vi "4 probe data v1.1.vi"() -> ()   [LabVIEW 2014]
uses:
  <vilib>/Analysis/baseanly.llb/Mean (DBL).vi
  <vilib>/MakerHub/LINX/Public/Peripherals/Analog/Analog Read 1 Chan.vi
  <instrlib>/Tektronix TDS 200 1000 2000 Series/Tektronix TDS 200 1000 2000 Series.lvlib
  <vilib>/MakerHub/LINX/LMH-LINX.lvlib
  <vilib>/Analysis/NI_AALBase.lvlib
panel:
  out "Data":string
  in  "Save File":path=path "c:/myfile.txt"
  out "Wavelength-Intensity Graph":cluster{"Y":dbl[], "Y":dbl[]}[](graph)
  out "Ch1 2":waveform(dbl)[](graph)
  out "Ch2 2":waveform(dbl)[](graph)
  out "Ch3 2":waveform(dbl)[](graph)
  out "Ch4 2":waveform(dbl)[](graph)
  out "Ch1":dbl
  out "Ch2":dbl
  out "Ch3":dbl
  out "Ch4":dbl
  out "Analog Data 0":dbl(graph)
  out "Loop Rate (Hz)":u32
  out "Analog Data 1":dbl(graph)
  out "Analog Data 2":dbl(graph)
  out "Analog Data 3":dbl(graph)
  out "Analog Data 4":dbl(graph)
  out "Numeric":dbl
  in  "AI Channel 4":u8
  in  "AI Channel 3":u8
  in  "AI Channel 2":u8
  in  "AI Channel 1":u8
  in  "AI Channel 0":u8
  in  "Serial Port":refnum<visa-resource-name>
  in  "Channel 4 (3: Channel 4)":u16(ring) items=["Channel 1", "Channel 2", "Channel 3", "Channel 4", "Math", "Reference A", "Reference B", "Reference C", "Reference D"]
  in  "Probe Attenuation 4 (0.1)":dbl=10.0
  in  "Vertical Coupling 4 (1: DC)":u16(ring)=1 items=["AC", "DC", "Ground"]
  in  "Channel 3 (2: Channel 3)":u16(ring) items=["Channel 1", "Channel 2", "Channel 3", "Channel 4", "Math", "Reference A", "Reference B", "Reference C", "Reference D"]
  in  "Probe Attenuation 3 (0.1)":dbl=10.0
  in  "Vertical Coupling 3 (1: DC)":u16(ring)=1 items=["AC", "DC", "Ground"]
  in  "Channel 2 (1: Channel 2)":u16(ring)=1 items=["Channel 1", "Channel 2", "Channel 3", "Channel 4", "Math", "Reference A", "Reference B", "Reference C", "Reference D"]
  in  "Channel 1 (0: Channel 1)":u16(ring) items=["Channel 1", "Channel 2", "Channel 3", "Channel 4", "Math", "Reference A", "Reference B", "Reference C", "Reference D"]
  in  "Serial Configuration":T1={"Baud Rate"=9600, "Parity"=0, "Stop Bits"=10, "Flow Control"=2} {"Flow Control" items=["None", "XON/XOFF", "RTS/CTS", "XON/XOFF & RTS/CTS", "DTR/DSR", "XON/XOFF & DTR/DSR"]; "Stop Bits" items=["1.0"=10, "1.5"=15, "2.0"=20]; "Parity" items=["None", "Odd", "Even", "Mark", "Space"]; "Baud Rate" items=["300"=300, "600"=600, "1200"=1200, "2400"=2400, "4800"=4800, "9600"=9600, "19200"=19200]}
  in  "Probe Attenuation 2 (0.1)":dbl=1.0
  in  "Vertical Coupling 2 (1: DC)":u16(ring)=1 items=["AC", "DC", "Ground"]
  in  "Probe Attenuation 1 (0.1)":dbl=10.0
  in  "Vertical Coupling 1 (1: DC)":u16(ring)=1 items=["AC", "DC", "Ground"]
  in  "Timeout (10000 ms)":u32=10000
  in  "VISA resource name":refnum<visa-resource-name>
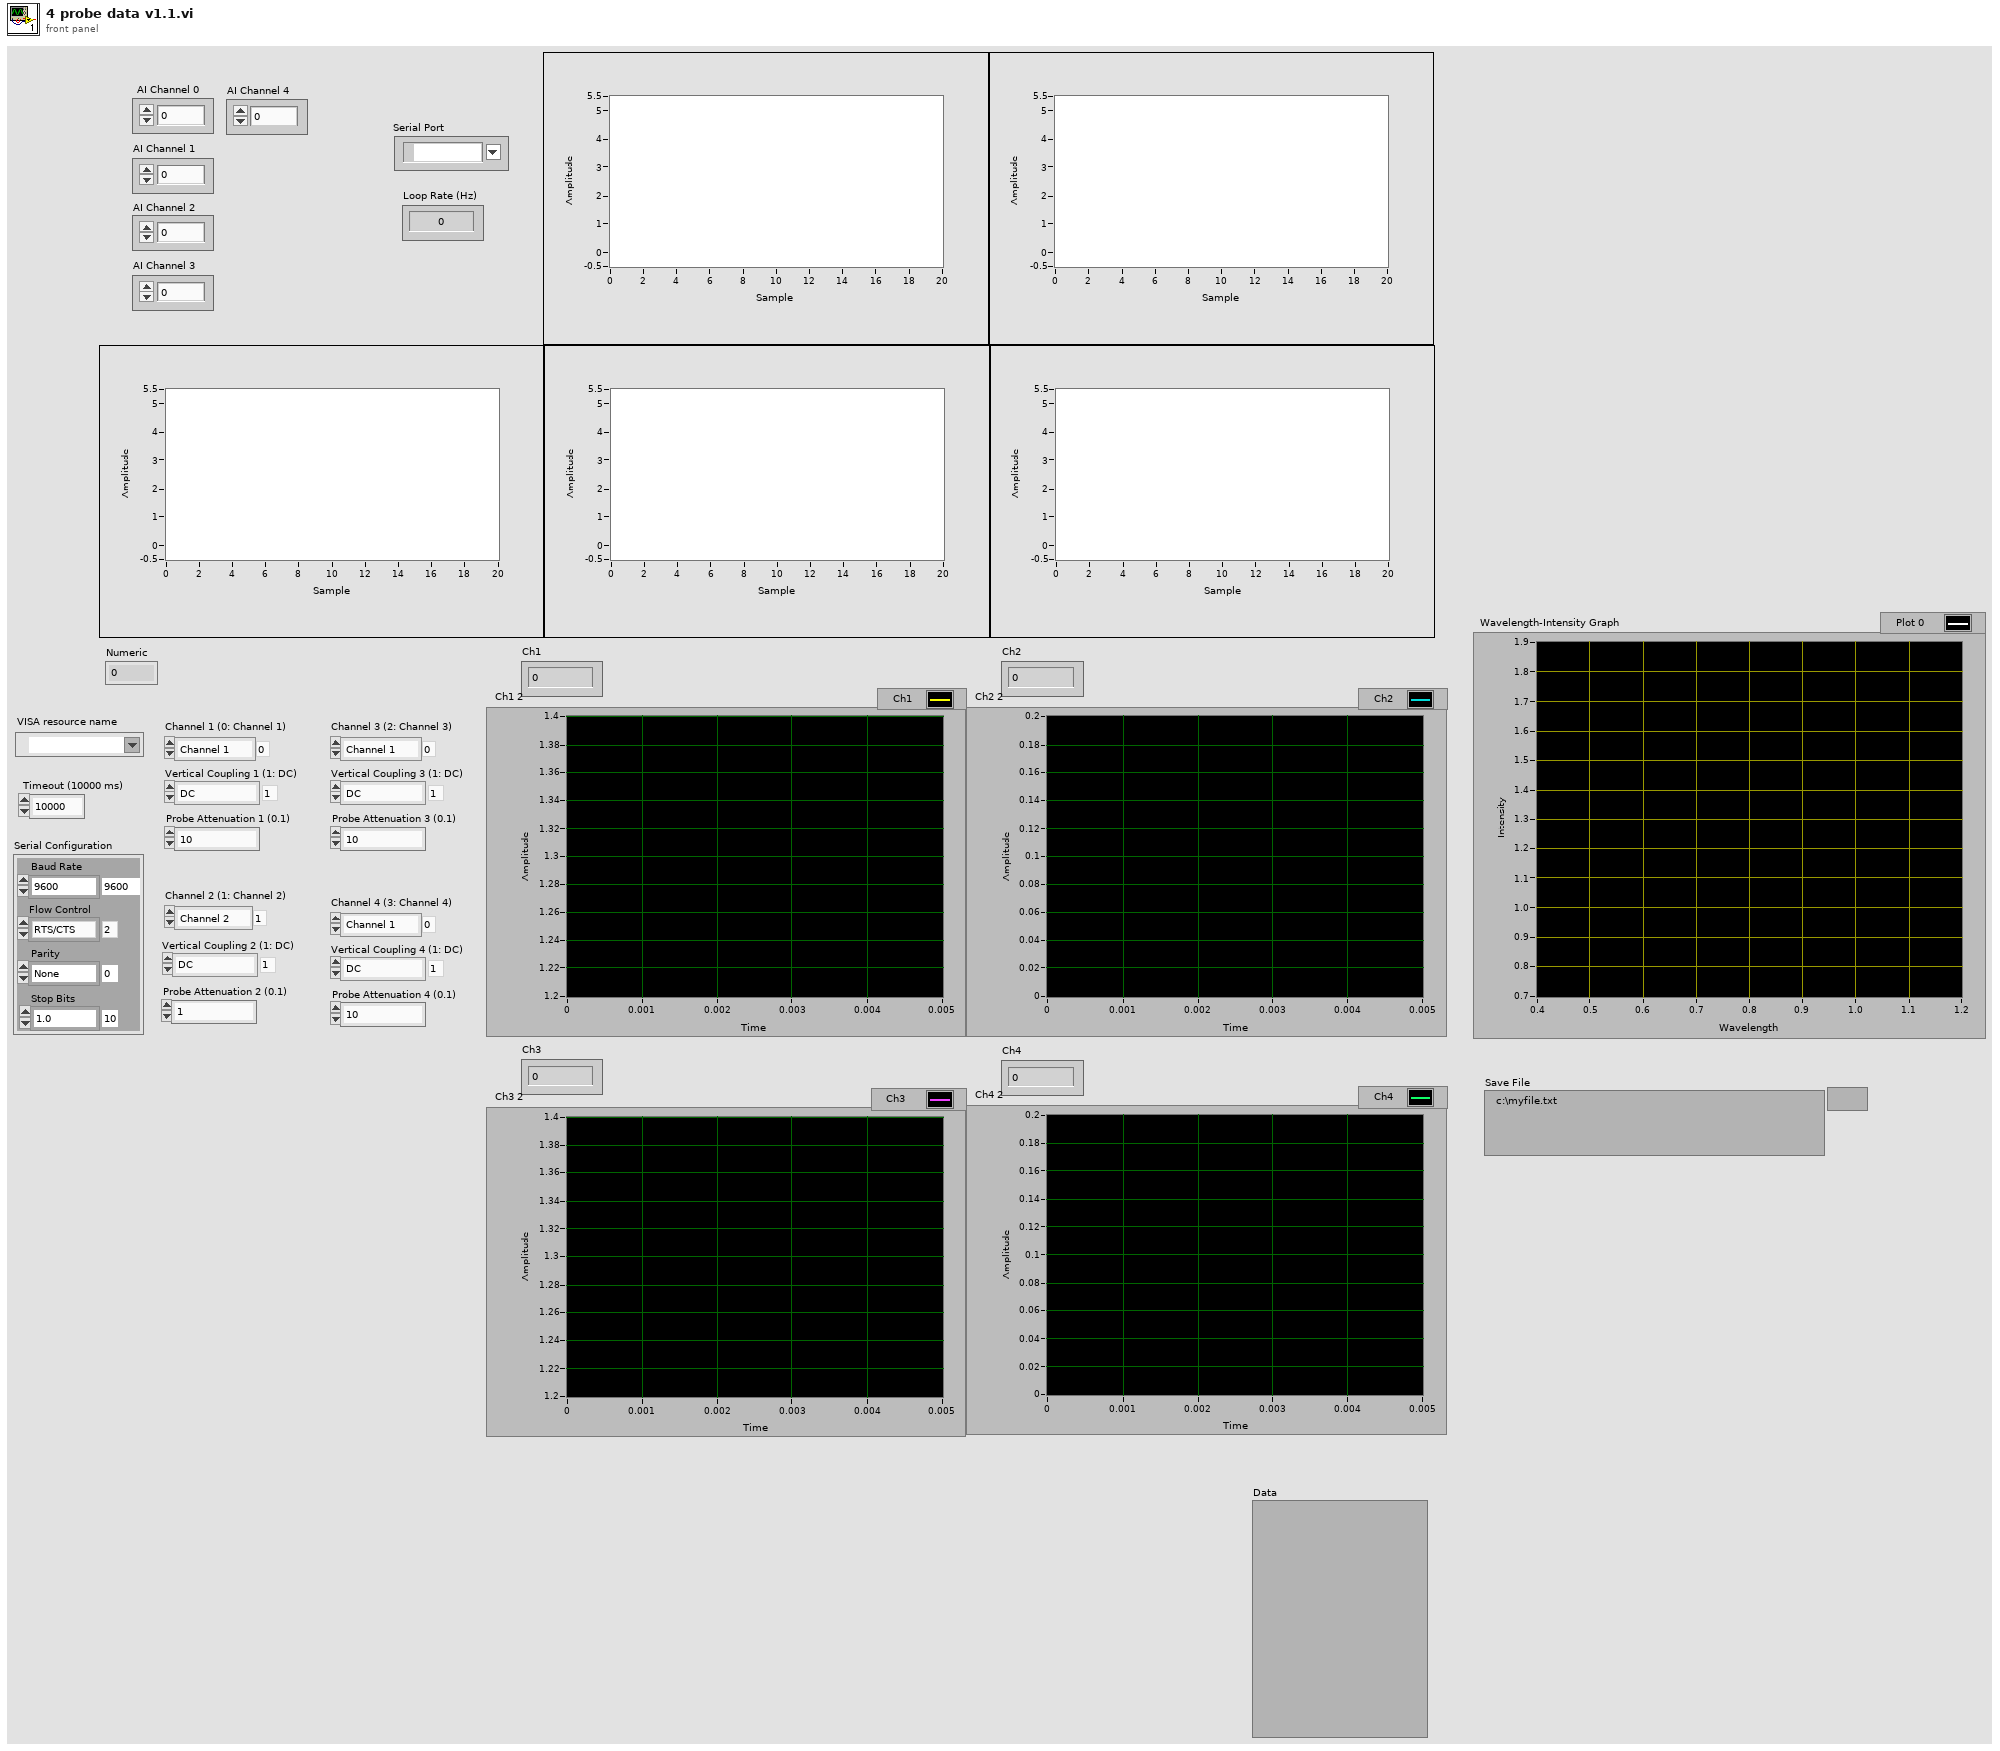
[diagram p1: front panel]
types:
  T1 = cluster{"Baud Rate":u32, "Parity":u16, "Stop Bits":u16, "Flow Control":u16}
  T2 = typedef "LMH-LINX.lvlib/LINX Ref.ctl" = cluster{"Platform":T3, "Interface":T4, "LINX Device Config":T5}
  T3 = typedef "LMH-LINX.lvlib/Platform.ctl" = enum16{"LINX", "myRIO"}
  T4 = typedef "LMH-LINX.lvlib/Interface.ctl" = enum16{"Serial", "TCP"}
  T5 = typedef "LMH-LINX.lvlib/Device.lvlib/LINX Device Config.ctl" = cluster{"Interface":T4, "COM Port":refnum<visa-resource-name>, "TCP Configuration":T6, "Device Family":u8, "Device ID":u8, "Device Name":string, "TCP Ref":refnum<k5>, "Channels":T7}
  T6 = typedef "LMH-LINX.lvlib/Device.lvlib/TCP Config.ctl" = cluster{"IP Address":string, "Port":u16}
  T7 = typedef "LMH-LINX.lvlib/Channels.ctl" = cluster{"DI":u8[], "DO":u8[], "AI":u8[], "AO":u8[], "PWM":u8[], "QE":u8[], "UART":u8[], "I2C 2":u8[], "SPI":u8[], "CAN":u8[], "Servo":u8[], "AI Ref (V)":dbl, "AO Ref (V)":dbl, "AO Resolution (Bits)":u8}
  T8 = enum16{"open", "replace", "create", "open or create", "replace or create", "replace or create with confirmation"}
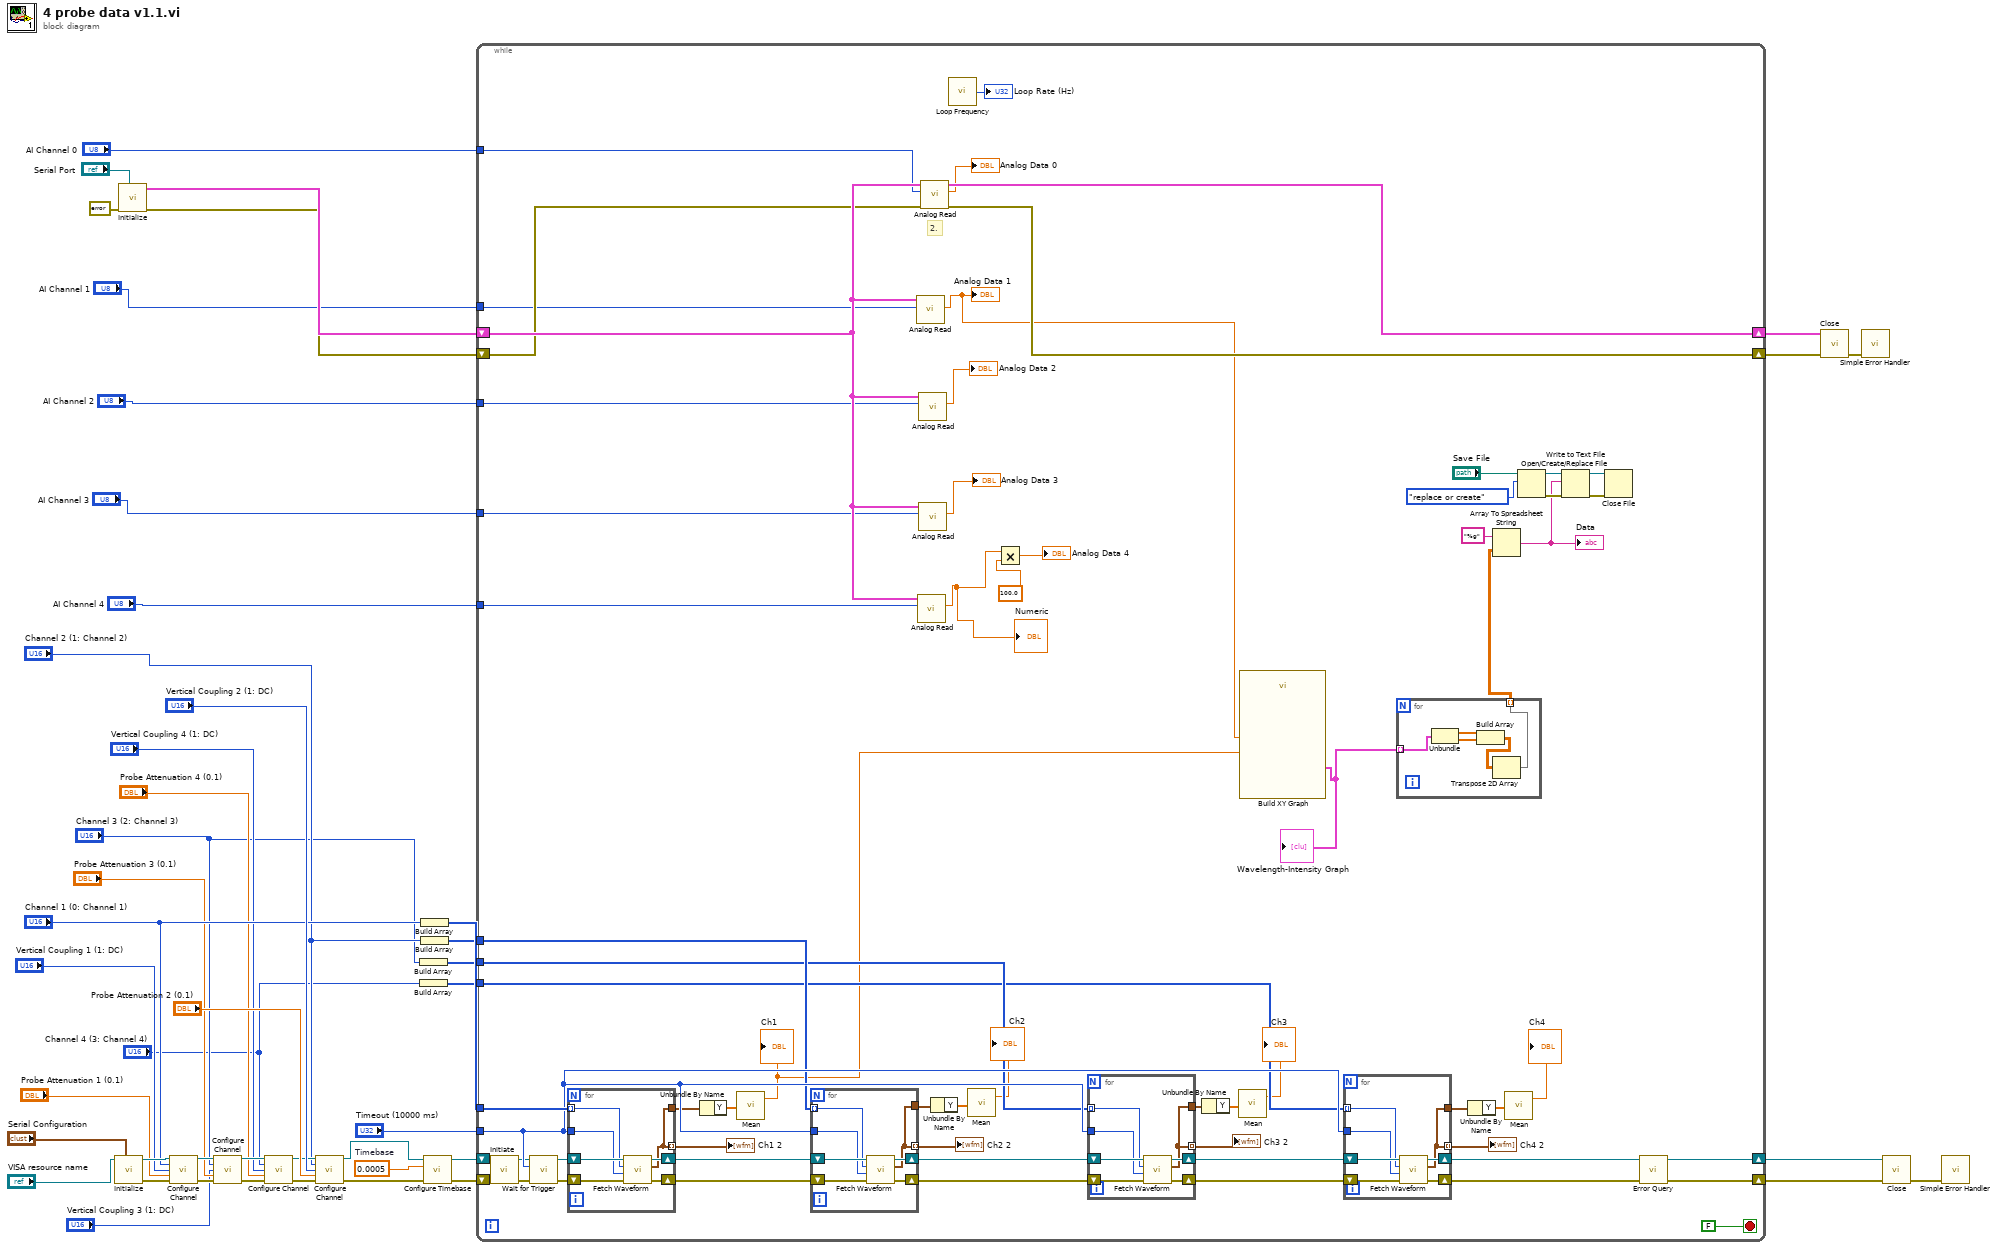
[diagram p0: block diagram]
diagram:
  w33 = 0.0005  # Timebase
  n1 = call <vilib>:"Initialize.vi"("Serial Configuration"="Serial Configuration", "VISA resource name"="VISA resource name") -> ("error out"=w42:errorcluster, "VISA resource name out"=w43:refnum<visa-resource-name>)  [unwired: 3 in, 5 out]
  n2 = call <vilib>:"Initialize.vi"("Serial Port"="Serial Port", "Error In"=errorcluster {"status"=FALSE, "code"=0, "source"=""}) -> ("Error Out"=w11:errorcluster, "LINX Ref"=w12:T2)  [unwired: 7 in, 1 out]
  n3 = call <instrlib>:"Configure Channel.vi"("VISA resource name"=w43, "Channel (0: Channel 1)"="Channel 1 (0: Channel 1)", "Vertical Coupling (1: DC)"="Vertical Coupling 1 (1: DC)", "Probe Attenuation (10: 10X)"="Probe Attenuation 1 (0.1)", "error in (no error)"=w42) -> ("VISA resource name out"=w28:refnum<visa-resource-name>, "error out"=w25:errorcluster)  [unwired: 4 in, 5 out]
  n4 = call <instrlib>:"Configure Channel.vi"("VISA resource name"=w28, "Channel (0: Channel 1)"="Channel 3 (2: Channel 3)", "Vertical Coupling (1: DC)"="Vertical Coupling 3 (1: DC)", "Probe Attenuation (10: 10X)"="Probe Attenuation 3 (0.1)", "error in (no error)"=w25) -> ("VISA resource name out"=w27:refnum<visa-resource-name>, "error out"=w24:errorcluster)  [unwired: 4 in, 5 out]
  n5 = call <instrlib>:"Configure Channel.vi"("VISA resource name"=w27, "Channel (0: Channel 1)"="Channel 4 (3: Channel 4)", "Vertical Coupling (1: DC)"="Vertical Coupling 4 (1: DC)", "Probe Attenuation (10: 10X)"="Probe Attenuation 4 (0.1)", "error in (no error)"=w24) -> ("VISA resource name out"=w26:refnum<visa-resource-name>, "error out"=w23:errorcluster)  [unwired: 4 in, 5 out]
  n6 = call <instrlib>:"Configure Channel.vi"("VISA resource name"=w26, "Channel (0: Channel 1)"="Channel 2 (1: Channel 2)", "Vertical Coupling (1: DC)"="Vertical Coupling 2 (1: DC)", "Probe Attenuation (10: 10X)"="Probe Attenuation 2 (0.1)", "error in (no error)"=w23) -> ("VISA resource name out"=w41:refnum<visa-resource-name>, "error out"=w40:errorcluster)  [unwired: 4 in, 5 out]
  n7 = Build Array("Channel 3 (2: Channel 3)") -> (w14:u16[])
  n8 = Build Array("Channel 4 (3: Channel 4)") -> (w13:u16[])
  n9 = Build Array("Channel 1 (0: Channel 1)") -> (w32:u16[])
  n10 = Build Array("Channel 2 (1: Channel 2)") -> (w17:u16[])
  n11 = call <instrlib>:"Configure Timebase.vi"("error in (no error)"=w40, "Timebase (0.0005 s)"=w33, "VISA resource name"=w41) -> ("error out"=w38:errorcluster, "VISA resource name out"=w39:refnum<visa-resource-name>)  [unwired: 1 in, 6 out]
  n12 = while {
    tunnel: w32 -> [w108]
    tunnel: "Timeout (10000 ms)" -> [w107]
    tunnel: w17 -> [w106]
    tunnel: w14 -> [w105]
    tunnel: w13 -> [w104]
    tunnel: "AI Channel 0" -> [w72]
    tunnel: "AI Channel 1" -> [w71]
    tunnel: "AI Channel 2" -> [w70]
    tunnel: "AI Channel 3" -> [w69]
    tunnel: "AI Channel 4" -> [w68]
    shift-right: [w112] -> w45
    shift-left: w39 -> [w110]
    shift-right: [w111] -> w44
    shift-left: w38 -> [w109]
    shift-right: [w74] -> w10
    shift-left: w12 -> [w76]
    shift-right: [w73] -> w9
    shift-left: w11 -> [w75]
    stop <- FALSE stop-if-true
    # "2."
    n13 = call <instrlib>:"Initiate.vi"("error in (no error)"=w109, "VISA resource name"=w110) -> ("error out"=w100:errorcluster, "VISA resource name out"=w103:refnum<visa-resource-name>)  [unwired: 8 out]
    n14 = call <instrlib>:"Wait for Trigger.vi"("error in (no error)"=w100, "Timeout (10000 ms)"=w107, "VISA resource name"=w103) -> ("error out"=w101:errorcluster, "VISA resource name out"=w102:refnum<visa-resource-name>)  [unwired: 7 out]
    n15 = for {
      shift-right: [w144] -> w97
      shift-left: w101 -> [w142]
      tunnel: w108 -> [w140] mode=indexing
      tunnel: [w139] -> w99 mode=indexing
      tunnel: w107 -> [w141]
      shift-right: [w145] -> w98
      shift-left: w102 -> [w143]
      tunnel: [w139] -> w87
      n16 = call <instrlib>:"Fetch Waveform.vi"("error in (no error)"=w142, "Timeout (10000 ms)"=w141, "Source (0: Channel 1)"=w140, "VISA resource name"=w143) -> ("error out"=w144:errorcluster, "Waveform Data"=w139:waveform(dbl), "VISA resource name out"=w145:refnum<visa-resource-name>)  [unwired: 2 in, 3 out]
    }
    "Ch1 2" <- w99
    n17 = Unbundle By Name(w87) -> ("Y"=w86:dbl[])
    n18 = call-poly <vilib>:"Mean.vi"("X"=w86) -> ("mean"=w49:dbl)  [unwired: 1 out]
    "Ch1" <- w49
    n19 = for {
      shift-right: [w137] -> w88
      shift-left: w97 -> [w135]
      tunnel: w106 -> [w133] mode=indexing
      tunnel: [w132] -> w96 mode=indexing
      tunnel: w107 -> [w134]
      shift-right: [w138] -> w89
      shift-left: w98 -> [w136]
      tunnel: [w132] -> w80
      n20 = call <instrlib>:"Fetch Waveform.vi"("error in (no error)"=w135, "Timeout (10000 ms)"=w134, "Source (0: Channel 1)"=w133, "VISA resource name"=w136) -> ("error out"=w137:errorcluster, "Waveform Data"=w132:waveform(dbl), "VISA resource name out"=w138:refnum<visa-resource-name>)  [unwired: 2 in, 3 out]
    }
    "Ch2 2" <- w96
    n21 = call-poly <vilib>:"Analog Read.vi"("Analog Channel"=w71, "LINX Resource"=w76) -> ("AI Value"=w48:dbl)  [unwired: 6 in, 3 out]
    "Analog Data 1" <- w48
    n22 = call-poly <vilib>:"Analog Read.vi"("Analog Channel"=w68, "LINX Resource"=w76) -> ("AI Value"=w62:dbl)  [unwired: 6 in, 3 out]
    "Numeric" <- w62
    n23 = call-poly <vilib>:"Analog Read.vi"("Analog Channel"=w70, "LINX Resource"=w76) -> ("AI Value"=→"Analog Data 2":dbl)  [unwired: 6 in, 3 out]
    n24 = call-poly <vilib>:"Analog Read.vi"("Analog Channel"=w69, "LINX Resource"=w76) -> ("AI Value"=→"Analog Data 3":dbl)  [unwired: 6 in, 3 out]
    n25 = call-poly <vilib>:"Analog Read.vi"("Error In"=w75, "Analog Channel"=w72, "LINX Resource"=w76) -> ("Error Out"=w73:errorcluster, "AI Value"=→"Analog Data 0":dbl, "LINX Resource"=w74:T2)  [unwired: 5 in, 1 out]
    n26 = Unbundle By Name(w80) -> ("Y"=w79:dbl[])
    n27 = call <vilib>:"Loop Frequency.vi"() -> ("Loop Rate (Hz)"=→"Loop Rate (Hz)":u32)
    n28 = call-poly <vilib>:"Mean.vi"("X"=w79) -> ("mean"=→"Ch2":dbl)  [unwired: 1 out]
    n29 = Multiply(x=w62, y=100.0) -> (x*y=→"Analog Data 4":dbl)
    n30 = for {
      shift-right: [w130] -> w92
      shift-left: w88 -> [w128]
      tunnel: w105 -> [w126] mode=indexing
      tunnel: [w125] -> w95 mode=indexing
      tunnel: w107 -> [w127]
      shift-right: [w131] -> w93
      shift-left: w89 -> [w129]
      tunnel: [w125] -> w81
      n31 = call <instrlib>:"Fetch Waveform.vi"("error in (no error)"=w128, "Timeout (10000 ms)"=w127, "Source (0: Channel 1)"=w126, "VISA resource name"=w129) -> ("error out"=w130:errorcluster, "Waveform Data"=w125:waveform(dbl), "VISA resource name out"=w131:refnum<visa-resource-name>)  [unwired: 2 in, 3 out]
    }
    "Ch3 2" <- w95
    n32 = Unbundle By Name(w81) -> ("Y"=w78:dbl[])
    n33 = call-poly <vilib>:"Mean.vi"("X"=w78) -> ("mean"=→"Ch3":dbl)  [unwired: 1 out]
    n34 = call "Build XY Graph"("Y Input"=w49, "X Input"=w48) -> ("XY Graph"=w50:cluster{"Y":dbl[], "Y":dbl[]}[])  [unwired: 8 in, 1 out]
    "Wavelength-Intensity Graph" <- w50
    n35 = for {
      shift-right: [w123] -> w90
      shift-left: w92 -> [w121]
      tunnel: w104 -> [w119] mode=indexing
      tunnel: [w118] -> w94 mode=indexing
      tunnel: w107 -> [w120]
      shift-right: [w124] -> w91
      shift-left: w93 -> [w122]
      tunnel: [w118] -> w82
      n36 = call <instrlib>:"Fetch Waveform.vi"("error in (no error)"=w121, "Timeout (10000 ms)"=w120, "Source (0: Channel 1)"=w119, "VISA resource name"=w122) -> ("error out"=w123:errorcluster, "Waveform Data"=w118:waveform(dbl), "VISA resource name out"=w124:refnum<visa-resource-name>)  [unwired: 2 in, 3 out]
    }
    "Ch4 2" <- w94
    n37 = for {
      tunnel: w50 -> [w117] mode=indexing
      tunnel: [w113] -> w51 mode=indexing
      n38 = Unbundle(w117) -> ("Y"=w116:dbl[], "Y"=w115:dbl[])
      n39 = Build Array(w116, w115) -> (w114:dbl[][])
      n40 = Transpose 2D Array(2D array=w114) -> (transposed array=w113:dbl[][])
    }
    n41 = Unbundle By Name(w82) -> ("Y"=w77:dbl[])
    n42 = Array To Spreadsheet String(array=w51, 3:"%g" ("format string")) -> (spreadsheet string=w52:string)  [unwired: 1 in]
    "Data" <- w52
    n43 = call-poly <vilib>:"Mean.vi"("X"=w77) -> ("mean"=→"Ch4":dbl)  [unwired: 1 out]
    n44 = Open/Create/Replace File(file path (use dialog)="Save File", operation (0:open)=T8."replace or create") -> (refnum out=w54:refnum<file>, error out=w59:errorcluster)  [unwired: 4 in, 1 out]
    n45 = Write to Text File(file (use dialog)=w54, text=w52, error in=w59) -> (refnum out=w57:refnum<file>, error out=w58:errorcluster)  [unwired: 2 out]
    n46 = Close File(refnum=w57, error in=w58) -> ()  [unwired: 2 out]
    n47 = call <instrlib>:"Error Query.vi"("error in (no error)"=w90, "VISA resource name"=w91) -> ("error out"=w111:errorcluster, "VISA resource name out"=w112:refnum<visa-resource-name>)  [unwired: 8 out]
  }
  n48 = call <instrlib>:"Close.vi"("Error In"=w9, "LINX Resource"=w10) -> ("Error Out"=w7:errorcluster)  [unwired: 8 in, 1 out]
  n49 = call <vilib>:"Simple Error Handler.vi"("error in (no error)"=w7) -> ()  [unwired: 4 in, 5 out]
  n50 = call <instrlib>:"Close.vi"("error in (no error)"=w44, "VISA resource name"=w45) -> ("error out"=w46:errorcluster)  [unwired: 9 out]
  n51 = call <vilib>:"Simple Error Handler.vi"("error in (no error)"=w46) -> ()  [unwired: 1 in, 8 out]
